vi "CAN Rate Calculator.vi"(11 "Baud Rate":u32=1000000) -> (2 "Max Frame Length":dbl[][](array[numeric]), 3 "Min Frame Length":dbl[][](array[numeric]))   [LabVIEW 2014, in "CAN Bus Monitor Engine.lvlib"]
uses:
  CAN Bus Monitor Engine.lvlib
panel:
  out "Bits Per Frame, Full Stuffing":u32
  out "Bits Per Frame, No Stuffing":u32
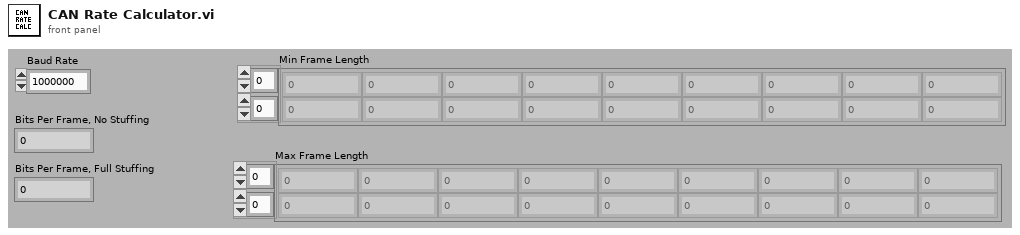
[diagram p1: front panel]
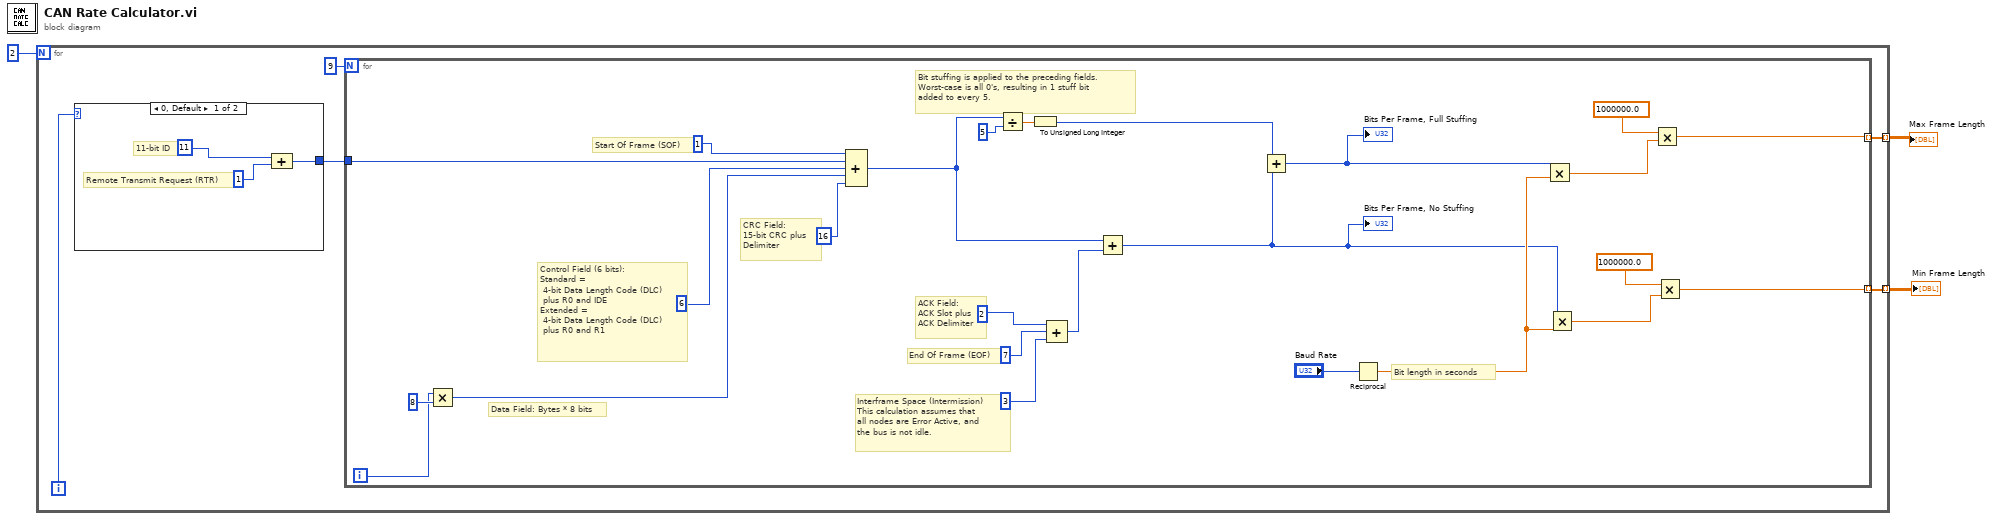
[diagram p0: block diagram]
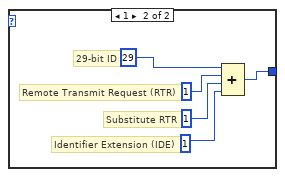
[diagram p2: hidden frame]
diagram:
  n1 = for {
    N: 2 -> [_]
    tunnel: [w5] -> w2 mode=indexing
    tunnel: [w4] -> w1 mode=indexing
    i -> [w7]
    n2 = case shown="0, Default" w7 {
      tunnel: [w34 w39] -> w8
      frame 0, Default {
        # "Remote Transmit Request (RTR)"
        # "11-bit ID"
        n3 = Compound Arithmetic op=unknown(11, 1) -> (w34:i32)
      }
      frame 1 {
        # "Identifier Extension (IDE)"
        # "Substitute RTR"
        # "Remote Transmit Request (RTR)"
        # "29-bit ID"
        n4 = Compound Arithmetic op=ADD(29, 1, 1, 1) -> (w39:i32)
      }
    }
    n5 = for {
      N: 9 -> [_]
      tunnel: w8 -> [w32]
      tunnel: [w9] -> w5 mode=indexing
      tunnel: [w10] -> w4 mode=indexing
      i -> [w11]
      # "Interframe Space (Intermission)\nThis calculation assumes that\nall nodes are Error Active, and\nthe bus is not idle."
      # "Bit length in seconds"
      # "End Of Frame (EOF)"
      # "ACK Field:\nACK Slot plus\nACK Delimiter"
      # "Bit stuffing is applied to the preceding fields.\nWorst-case is all 0's, resulting in 1 stuff bit\nadded to every 5."
      # "CRC Field:\n15-bit CRC plus \nDelimiter"
      # "Data Field: Bytes * 8 bits"
      # "Control Field (6 bits):\nStandard = \n 4-bit Data Length Code (DLC)\n plus R0 and IDE\nExtended = \n 4-bit Data Length Code (DLC)\n plus R0 and R1"
      # "Start Of Frame (SOF)"
      n6 = Multiply(x=w11, y=u32 8) -> (x*y=w29:u32)
      n7 = Compound Arithmetic op=ADD(1, w32, 6, w29, 16) -> (w23:u32)
      n8 = Divide(x=w23, y=u32 5) -> (x/y=w21:dbl)
      n9 = To Unsigned Long Integer(number=w21) -> (unsigned 32bit integer=w20:u32)
      n10 = Compound Arithmetic op=unknown(2, 7, 3) -> (w22:i32)
      n11 = Add(x=w23, y=w22) -> (x+y=w13:u32)
      "Bits Per Frame, No Stuffing" <- w13
      n12 = Add(x=w20, y=w13) -> (x+y=w12:u32)
      "Bits Per Frame, Full Stuffing" <- w12
      n13 = Reciprocal(x="Baud Rate") -> (1/x=w17:dbl)
      n14 = Multiply(x=w12, y=w17) -> (x*y=w14:dbl)
      n15 = Multiply(x=w13, y=w17) -> (x*y=w15:dbl)
      n16 = Multiply(x=1000000.0 ("y"), y=w14) -> (x*y=w9:dbl)
      n17 = Multiply(x=1000000.0 ("y"), y=w15) -> (x*y=w10:dbl)
    }
  }
  "Min Frame Length" <- w1
  "Max Frame Length" <- w2
